vi "test_Channels to Define (JSON RCT).vi"(8 "error in":errorcluster) -> (0 "error out":errorcluster)   [LabVIEW 2020, in "Test_Routing Templates.lvlib"]
uses:
  Test_Routing Templates.lvlib
  <vilib>/addons/_JKI Toolkits/Caraya/classes/Test/Test.lvclass
  <vilib>/addons/_JKI Toolkits/Caraya/classes/Assert/Assert.lvclass
  Routing Channel Templates/JSON Routing Channel Template/JSON Routing Channel Template.lvclass
  <vilib>/addons/_JKI Toolkits/Caraya/classes/Assert/Assert Equal Value_Variant.vi
  deaa77bd-6bfa-485a-96be-0d71bb0d6600.vi
  6b2e7e3b-8c53-4cba-bb39-c40b49200525.vi
  C:/Users/mjacobso/Desktop/SCM/Routing-Faulting/Source/Routing and Faulting/Routing Templates/Routing Channel Templates/Abstract Routing Channel Template/Abstract Routing Channel Template.lvclass
  C:/Users/mjacobso/Desktop/SCM/Routing-Faulting/Source/Routing and Faulting/Routing Templates/Routing Channel Templates/JSON Routing Channel Template/JSON Routing Channel Template.lvclass
  7ee95aeb-aa81-4ec0-9af3-663c7150f8b0.vi
  1b56ce28-15c7-451a-b51d-d960499f1d89.vi
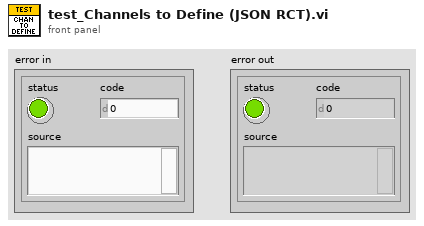
[diagram p1: front panel]
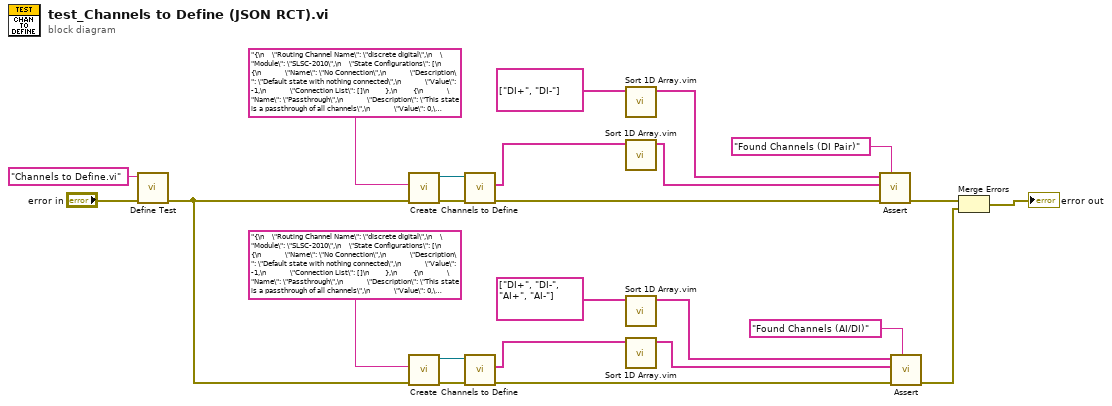
[diagram p0: block diagram]
diagram:
  n1 = call <vilib>:"Define Test.vi"("error in (no error)"="error in", "Label (VI Title)"="Channels to Define.vi") -> ("error out"=w10:errorcluster)  [unwired: 9 in]
  n2 = call "Create.vi"("error in (no error)"=w10, "JSON"="{\n    \"Routing Channel Name\": \"discrete digital\",\n    \"Module\": \"SLSC-2010\",\n    \"State Configurations\": [\n        {\n            \"Name\": \"No Connection\",\n            \"Description\": \"Default state with nothing connected\",\n            \"Value\": -1,\n            \"Connection List\": []\n        },\n        {\n            \"Name\": \"Passthrough\",\n            \"Description\": \"This state is a passthrough of all channels\",\n            \"Value\": 0,\n            \"Connection List\": [\n                {\n                    \"Channel\": \"DI+\",\n                    \"Connection Type\": \"Passthrough\"\n                },\n                {\n                    \"Channel\": \"DI-\",\n                    \"Connection Type\": \"Passthrough\"\n                }\n            ]\n        },\n        {\n            \"Name\": \"Real-Sim\",\n            \"Description\": \"Connect J1 to J2 pins\",\n            \"Value\": 1,\n            \"Connection List\": [\n                {\n                    \"Channel\": \"DI+\",\n                    \"Connection Type\": \"Real-Sim\"\n                },\n                {\n                    \"Channel\": \"DI-\",\n                    \"Connection Type\": \"Real-Sim\"\n                }\n            ]\n        }\n    ]\n}" ("text")) -> ("error out"=w17:errorcluster, "JSON Routing Channel Template out"=w18:refnum<class "JSON Routing Channel Template.lvclass">)  [unwired: 8 in]
  n3 = call "Create.vi"("error in (no error)"=w10, "JSON"="{\n    \"Routing Channel Name\": \"discrete digital\",\n    \"Module\": \"SLSC-2010\",\n    \"State Configurations\": [\n        {\n            \"Name\": \"No Connection\",\n            \"Description\": \"Default state with nothing connected\",\n            \"Value\": -1,\n            \"Connection List\": []\n        },\n        {\n            \"Name\": \"Passthrough\",\n            \"Description\": \"This state is a passthrough of all channels\",\n            \"Value\": 0,\n            \"Connection List\": [\n                {\n                    \"Channel\": \"AI+\",\n                    \"Connection Type\": \"Passthrough\"\n                },\n                {\n                    \"Channel\": \"AI-\",\n                    \"Connection Type\": \"Passthrough\"\n                }\n            ]\n        },\n        {\n            \"Name\": \"Real-Sim\",\n            \"Description\": \"Connect J1 to J2 pins\",\n            \"Value\": 1,\n            \"Connection List\": [\n                {\n                    \"Channel\": \"DI+\",\n                    \"Connection Type\": \"Real-Sim\"\n                },\n                {\n                    \"Channel\": \"DI-\",\n                    \"Connection Type\": \"Real-Sim\"\n                }\n            ]\n        }\n    ]\n}" ("text")) -> ("error out"=w14:errorcluster, "JSON Routing Channel Template out"=w13:refnum<class "JSON Routing Channel Template.lvclass">)  [unwired: 8 in]
  n4 = call-dynamic "Channels to Define.vi"("error in (no error)"=w17, "JSON Routing Channel Template in"=w18) -> ("error out"=w16:errorcluster, "Channels"=w3:string[])  [unwired: 7 in, 1 out]
  n5 = call-dynamic "Channels to Define.vi"("error in (no error)"=w14, "JSON Routing Channel Template in"=w13) -> ("error out"=w15:errorcluster, "Channels"=w7:string[])  [unwired: 7 in, 1 out]
  n6 = call "Sort 1D Array.vim"("unsorted array"=string[] ["DI+", "DI-"] ("Channels")) -> ("sorted array"=w1:string[])  [unwired: 10 in]
  n7 = call "Sort 1D Array.vim"("unsorted array"=w3) -> ("sorted array"=w2:string[])  [unwired: 10 in]
  n8 = call "Sort 1D Array.vim"("unsorted array"=string[] ["DI+", "DI-", "AI+", "AI-"] ("Channels")) -> ("sorted array"=w5:string[])  [unwired: 10 in]
  n9 = call "Sort 1D Array.vim"("unsorted array"=w7) -> ("sorted array"=w6:string[])  [unwired: 10 in]
  n10 = call-poly <vilib>:"Assert.vi"("Label"="Found Channels (DI Pair)", "error in (no error)"=w16, "Y"=w2, "X"=w1) -> ("error out"=w22:errorcluster)  [unwired: 7 in]
  n11 = call-poly <vilib>:"Assert.vi"("Label"="Found Channels (AI/DI)", "error in (no error)"=w15, "Y"=w6, "X"=w5) -> ("error out"=w9:errorcluster)  [unwired: 7 in]
  n12 = Merge Errors(w22, w9) -> (→"error out":errorcluster)
